vi "ReadPropertyInTDMS.vi"(3 "数组":variant[](array[variant])) -> (1 "输出簇":T1)   [LabVIEW 2012]
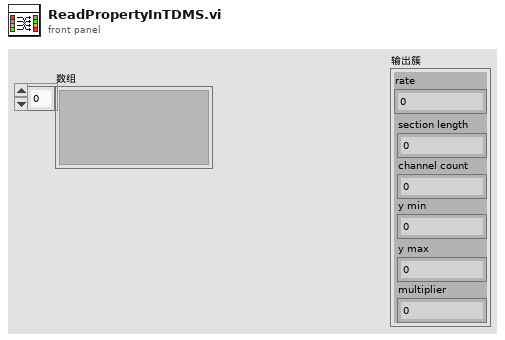
[diagram p1: front panel]
types:
  T1 = cluster{"rate":dbl, "section length":u32, "channel count":u32, "y min":dbl, "y max":dbl, "multiplier":dbl}
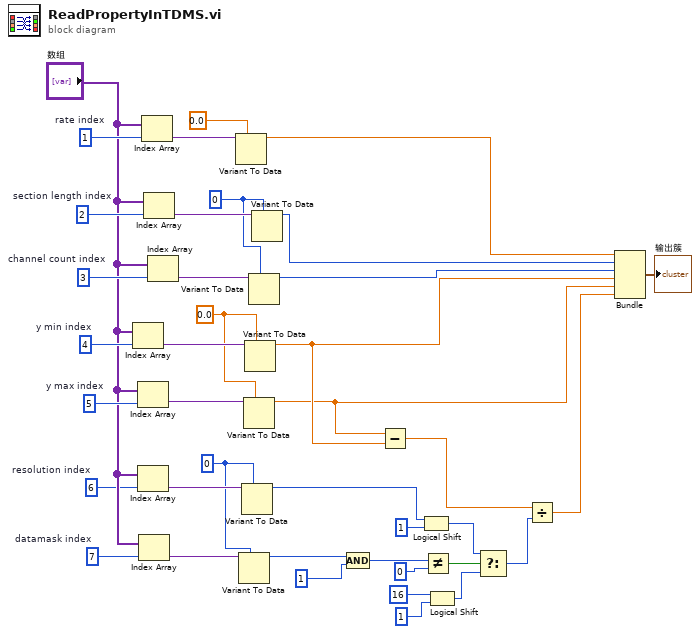
[diagram p0: block diagram]
diagram:
  w21 = 0
  w24 = 7  # datamask index
  w25 = 6  # resolution index
  w29 = u32 0
  w27 = 0.0
  w32 = 4  # y min index
  w33 = 5  # y max index
  w28 = 3  # channel count index
  w35 = u32 2  # section length index
  w39 = 1  # rate index
  n1 = Index Array(array="数组", index=w32) -> (element=w31:variant)
  n2 = Index Array(array="数组", index=w33) -> (element=w30:variant)
  n3 = Index Array(array="数组", index=w25) -> (element=w23:variant)
  n4 = Index Array(array="数组", index=w24) -> (element=w22:variant)
  n5 = Index Array(array="数组", index=w39) -> (element=w38:variant)
  n6 = Index Array(array="数组", index=w35) -> (element=w36:variant)
  n7 = Index Array(array="数组", index=w28) -> (element=w34:variant)
  n8 = Variant To Data(type=0.0, Variant=w38) -> (data=w7:dbl)  [unwired: 1 in, 1 out]
  n9 = Variant To Data(type=w21, Variant=w22) -> (data=w20:i32)  [unwired: 1 in, 1 out]
  n10 = Variant To Data(type=w21, Variant=w23) -> (data=w12:i32)  [unwired: 1 in, 1 out]
  n11 = Variant To Data(type=w27, Variant=w30) -> (data=w3:dbl)  [unwired: 1 in, 1 out]
  n12 = Variant To Data(type=w27, Variant=w31) -> (data=w4:dbl)  [unwired: 1 in, 1 out]
  n13 = Variant To Data(type=w29, Variant=w34) -> (data=w5:u32)  [unwired: 1 in, 1 out]
  n14 = Variant To Data(type=w29, Variant=w36) -> (data=w6:u32)  [unwired: 1 in, 1 out]
  n15 = Compound Arithmetic op=AND(w20, 1 ("值")) -> (w18:i32)
  n16 = Subtract(x=w3, y=w4) -> (x-y=w15:dbl)
  n17 = Logical Shift(y=w12, x=u64 1) -> (x << y=w9:u64)
  n18 = Not Equal?(x=w18, y=0) -> (x != y?=w16:bool)
  n19 = Logical Shift(y=i16 16, x=u64 1) -> (x << y=w8:u64)
  n20 = Select(t=w9, s=w16, f=w8) -> (s? t:f=w14:u64)
  n21 = Divide(x=w15, y=w14) -> (x/y=w2:dbl)
  n22 = Bundle(w7, w6, w5, w4, w3, w2) -> (→"输出簇":cluster{dbl, u32, u32, dbl, dbl, dbl})  [unwired: 1 in]
